vi "CH_States.vi"(8 "Error In":errorcluster, 9 "Channel No":T2=13 items=["7"=7, "11"=11, "12"=12, "13"=13, "15"=15, "16"=16, "18"=18, "29"=29, "32"=32, "33"=33, "35"=35, "36"=36, "37"=37, "38"=38, "40"=40], 10 "State":bool, 11 "CHStIn":T1) -> (0 "Error Out":errorcluster, 3 "CHStOut":T1)   [LabVIEW 2021, in "ValveCTRL.lvlib"]
uses:
  ValveCTRL.lvlib
  TypeDef/CHs_List.ctl
  TypeDef/ChannelStatus.ctl
  <vilib>/Utility/error.llb/Error Cluster From Error Code.vi
  <vilib>/ErrorRing/Error Ring.xnode
  Main/Main.lvlib
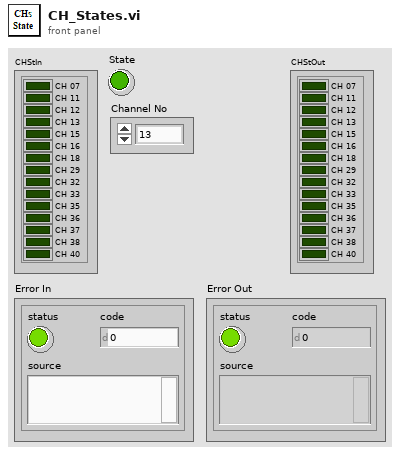
[diagram p1: front panel]
types:
  T1 = typedef "ValveCTRL.lvlib/ChannelStatus.ctl" = cluster{"CH 07":bool, "CH 11":bool, "CH 12":bool, "CH 13":bool, "CH 15":bool, "CH 16":bool, "CH 18":bool, "CH 29":bool, "CH 32":bool, "CH 33":bool, "CH 35":bool, "CH 36":bool, "CH 37":bool, "CH 38":bool, "CH 40":bool}
  T2 = typedef "ValveCTRL.lvlib/CHs_List.ctl" = u8
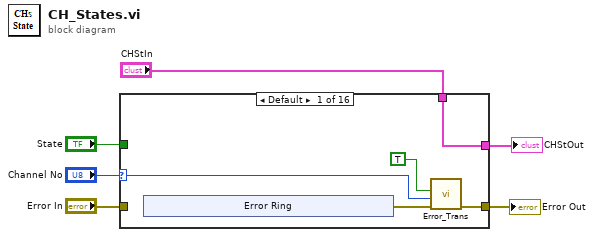
[diagram p0: block diagram]
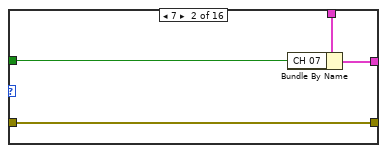
[diagram p2: hidden frame]
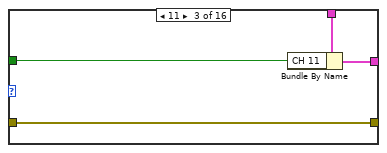
[diagram p3: hidden frame]
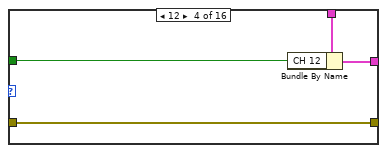
[diagram p4: hidden frame]
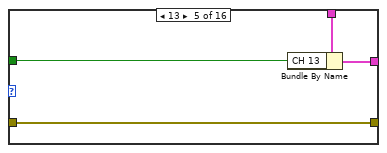
[diagram p5: hidden frame]
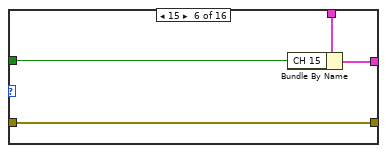
[diagram p6: hidden frame]
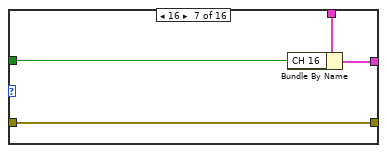
[diagram p7: hidden frame]
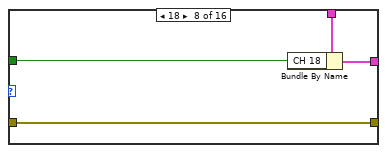
[diagram p8: hidden frame]
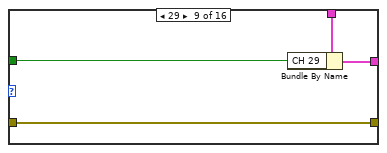
[diagram p9: hidden frame]
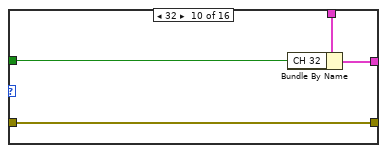
[diagram p10: hidden frame]
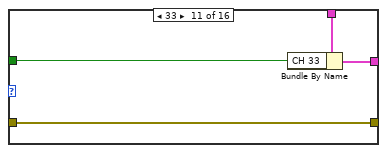
[diagram p11: hidden frame]
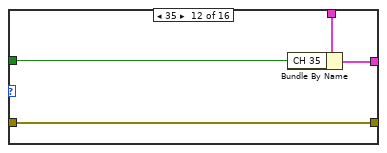
[diagram p12: hidden frame]
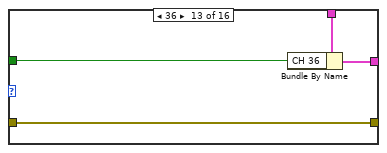
[diagram p13: hidden frame]
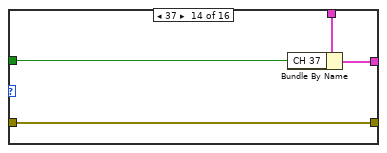
[diagram p14: hidden frame]
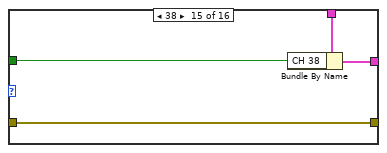
[diagram p15: hidden frame]
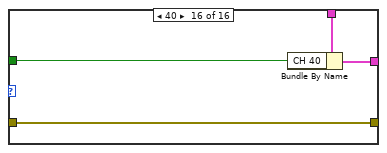
[diagram p16: hidden frame]
diagram:
  n1 = case shown="Default" "Channel No" {
    selector: "Channel No" -> [w8 _ _ _ _ _ _ _ _ _ _ _ _ _ _ _]
    tunnel: "State" -> [_ w18 w22 w26 w30 w34 w38 w42 w46 w50 w54 w58 w62 w66 w70 w74]
    tunnel: "CHStIn" -> [w11 w19 w23 w27 w31 w35 w39 w43 w47 w51 w55 w59 w63 w67 w71 w75]
    tunnel: [w11 w17 w21 w25 w29 w33 w37 w41 w45 w49 w53 w57 w61 w65 w69 w73] -> w3
    tunnel: "Error In" -> [_ w16 w20 w24 w28 w32 w36 w40 w44 w48 w52 w56 w60 w64 w68 w72]
    tunnel: [w9 w16 w20 w24 w28 w32 w36 w40 w44 w48 w52 w56 w60 w64 w68 w72] -> w1
    frame Default {
      n2 = xnode "Error Ring"() -> ("error out"=w10:errorcluster)
      n3 = call "Error_Trans.vi"("Error In"=w10, "VAR"=w8, "Add_s%"=TRUE) -> ("Error Out"=w9:errorcluster)  [unwired: 7 in, 1 out]
    }
    frame 7 {
      n4 = Bundle By Name(cluster=w19, "CH 07"=w18) -> (w17:T1)
    }
    frame 11 {
      n5 = Bundle By Name(cluster=w23, "CH 11"=w22) -> (w21:T1)
    }
    frame 12 {
      n6 = Bundle By Name(cluster=w27, "CH 12"=w26) -> (w25:T1)
    }
    frame 13 {
      n7 = Bundle By Name(cluster=w31, "CH 13"=w30) -> (w29:T1)
    }
    frame 15 {
      n8 = Bundle By Name(cluster=w35, "CH 15"=w34) -> (w33:T1)
    }
    frame 16 {
      n9 = Bundle By Name(cluster=w39, "CH 16"=w38) -> (w37:T1)
    }
    frame 18 {
      n10 = Bundle By Name(cluster=w43, "CH 18"=w42) -> (w41:T1)
    }
    frame 29 {
      n11 = Bundle By Name(cluster=w47, "CH 29"=w46) -> (w45:T1)
    }
    frame 32 {
      n12 = Bundle By Name(cluster=w51, "CH 32"=w50) -> (w49:T1)
    }
    frame 33 {
      n13 = Bundle By Name(cluster=w55, "CH 33"=w54) -> (w53:T1)
    }
    frame 35 {
      n14 = Bundle By Name(cluster=w59, "CH 35"=w58) -> (w57:T1)
    }
    frame 36 {
      n15 = Bundle By Name(cluster=w63, "CH 36"=w62) -> (w61:T1)
    }
    frame 37 {
      n16 = Bundle By Name(cluster=w67, "CH 37"=w66) -> (w65:T1)
    }
    frame 38 {
      n17 = Bundle By Name(cluster=w71, "CH 38"=w70) -> (w69:T1)
    }
    frame 40 {
      n18 = Bundle By Name(cluster=w75, "CH 40"=w74) -> (w73:T1)
    }
  }
  "CHStOut" <- w3
  "Error Out" <- w1
